vi "PosTransToCalib.vi"(10 "ToolData":cluster{"X":dbl, "Y":dbl, "Angle":dbl}, 11 "Vision&Robot":T1(array[cluster])) -> (2 "Real":cluster{"X":dbl, "Y":dbl}[](array[cluster]), 3 "Vision":cluster{"X":dbl, "Y":dbl}[](array[cluster]))   [LabVIEW 2019]
uses:
  <vilib>/Analysis/coordinate.llb/2D Cartesian Coordinate Rotation (Scalar).vi
  <vilib>/Analysis/NI_AALPro.lvlib
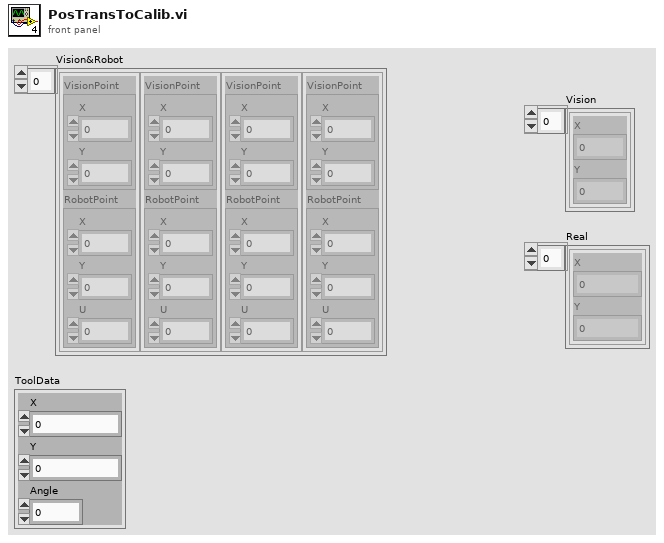
[diagram p1: front panel]
types:
  T1 = cluster{"VisionPoint":cluster{"X":dbl, "Y":dbl}, "RobotPoint":cluster{"X":dbl, "Y":dbl, "U":dbl}}[]
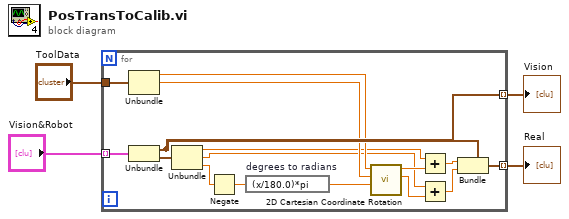
[diagram p0: block diagram]
diagram:
  n1 = for {
    tunnel: "Vision&Robot" -> [w20] mode=indexing
    tunnel: [w19] -> w1 mode=indexing
    tunnel: [w18] -> w2 mode=indexing
    tunnel: "ToolData" -> [w16]
    n2 = Unbundle(w16) -> ("X"=w15:dbl, "Y"=w14:dbl)  [unwired: 1 out]
    n3 = Unbundle(w20) -> ("VisionPoint"=w19:cluster{"X":dbl, "Y":dbl}, "RobotPoint"=w17:cluster{"X":dbl, "Y":dbl, "U":dbl})
    n4 = Unbundle(w17) -> ("X"=w13:dbl, "Y"=w10:dbl, "U"=w7:dbl)
    n5 = Negate(x=w7) -> (-x=w5:dbl)
    n6 = expression code="(x/180.0)*pi" "degrees to radians"(w5) -> (w6:dbl)
    n7 = call-poly <vilib>:"2D Cartesian Coordinate Rotation.vi"("theta"=w6, "y"=w14, "x"=w15) -> ("y out"=w9:dbl, "x out"=w12:dbl)  [unwired: 6 in, 1 out]
    n8 = Add(x=w13, y=w12) -> (x+y=w11:dbl)
    n9 = Add(x=w10, y=w9) -> (x+y=w8:dbl)
    n10 = Bundle(cluster=w19, "X"=w11, "Y"=w8) -> (w18:cluster{"X":dbl, "Y":dbl})
  }
  "Real" <- w2
  "Vision" <- w1
